vi "ArrayView.vi"(4 "Properties":T2={"Colormap"={"Map"=enum."Automatic", "Value Min"=nan, "Value Max"=nan, "Scaling"=enum."Default", "Reverse"=FALSE}, "Display"={"Alpha"=nan, "Z Order"=nan}}, 6 "Boundaries":T1={"X Min"=nan, "X Max"=nan, "Y Min"=nan, "Y Max"=nan}, 7 "Data":dbl[][](array[numeric]), 8 "error in (no error)":errorcluster, 11 "Plot ID":T7 format="%x") -> (0 "error out":errorcluster, 3 "Plot ID Out":T7 format="%x")   [LabVIEW 2013, in "Advanced Plotting Toolkit.lvlib"]
doc: "Display a 2D array as pseudocolor, using a colormap."
uses:
  Advanced Plotting Toolkit.lvlib
  typedefs/PlotID.ctl
  ArrayViewProperties.ctl
  properties/Colormap.ctl
  properties/Colormap_Map.ctl
  properties/Colormap_Scaling.ctl
  properties/Display.ctl
  ArrayViewBoundaries.ctl
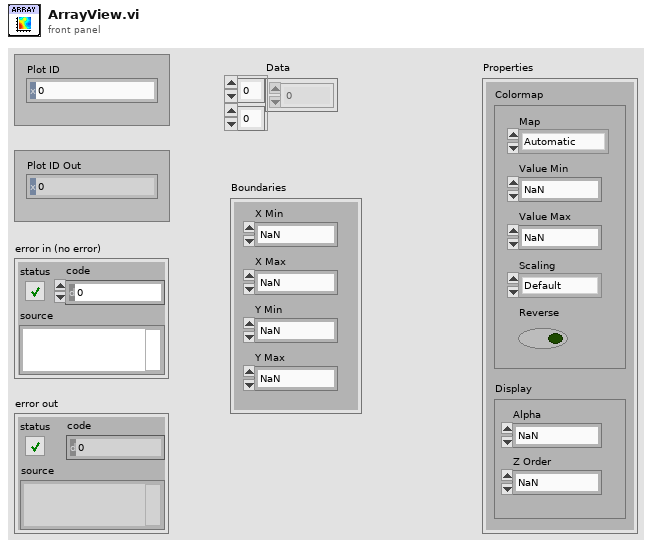
[diagram p1: front panel]
types:
  T1 = typedef "Advanced Plotting Toolkit.lvlib/ArrayViewBoundaries.ctl" = cluster{"X Min":dbl, "X Max":dbl, "Y Min":dbl, "Y Max":dbl}
  T2 = typedef "Advanced Plotting Toolkit.lvlib/ArrayViewProperties.ctl" = cluster{"Colormap":T3, "Display":T6}
  T3 = typedef "Advanced Plotting Toolkit.lvlib/Colormap.ctl" = cluster{"Map":T4, "Value Min":dbl, "Value Max":dbl, "Scaling":T5, "Reverse":bool}
  T4 = typedef "Advanced Plotting Toolkit.lvlib/Colormap_Map.ctl" = enum16{"Automatic", "Rainbow", "Hot and Cold", "White-Black", "White-Blue", "White-Green", "White-Red", "Fire", "Water", "Earth", "Air", "Pastel", "Banded", "Stepped"}
  T5 = typedef "Advanced Plotting Toolkit.lvlib/Colormap_Scaling.ctl" = enum16{"Default"}
  T6 = typedef "Advanced Plotting Toolkit.lvlib/Display.ctl" = cluster{"Alpha":dbl, "Z Order":dbl}
  T7 = typedef "Advanced Plotting Toolkit.lvlib/PlotID.ctl" = i32
  T8 = typedef "Advanced Plotting Toolkit.lvlib/KeyValue.ctl" = cluster{"Key":string, "Value":string}
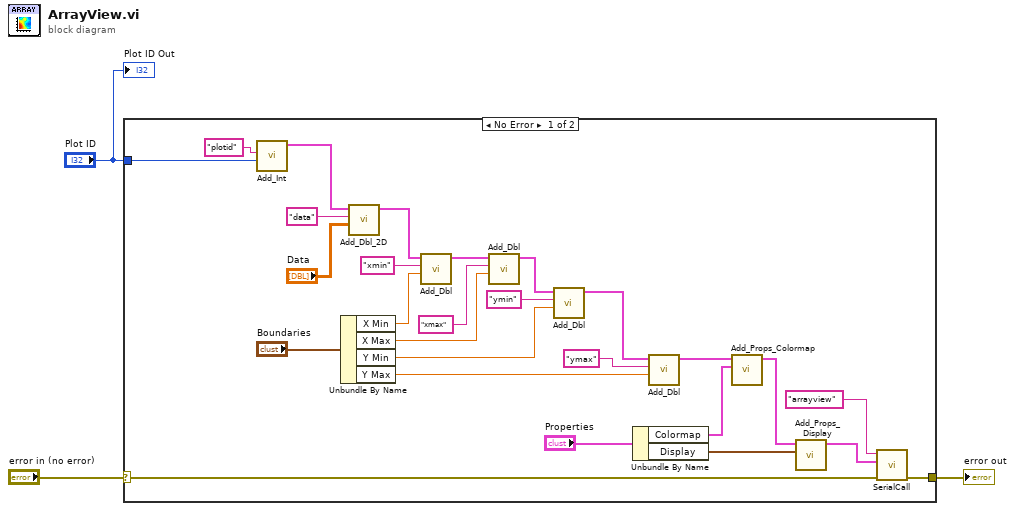
[diagram p0: block diagram]
diagram:
  n1 = case shown="No Error" "error in (no error)" {
    selector: "error in (no error)" -> [w28 w31]
    tunnel: "Plot ID" -> [w30 _]
    tunnel: [w27 w31] -> w1
    frame No Error {
      n2 = call "Add_Int.vi"("Value"=w30, "Key"="plotid") -> ("Keyword Array Out"=w26:T8[])  [unwired: 9 in]
      n3 = Unbundle By Name("Boundaries") -> ("X Min"=w7:dbl, "X Max"=w6:dbl, "Y Min"=w5:dbl, "Y Max"=w4:dbl)
      n4 = call "Add_Dbl_2D.vi"("Value"="Data", "Key"="data", "Keyword Array"=w26) -> ("Keyword Array Out"=w17:T8[])  [unwired: 8 in]
      n5 = call "Add_Dbl.vi"("Value"=w7, "Key"="xmin", "Keyword Array"=w17) -> ("Keyword Array Out"=w12:T8[])  [unwired: 8 in]
      n6 = call "Add_Dbl.vi"("Value"=w6, "Key"="xmax", "Keyword Array"=w12) -> ("Keyword Array Out"=w11:T8[])  [unwired: 8 in]
      n7 = call "Add_Dbl.vi"("Value"=w5, "Key"="ymin", "Keyword Array"=w11) -> ("Keyword Array Out"=w10:T8[])  [unwired: 8 in]
      n8 = Unbundle By Name("Properties") -> ("Colormap"=w22:T3, "Display"=w20:T6)
      n9 = call "Add_Dbl.vi"("Value"=w4, "Key"="ymax", "Keyword Array"=w10) -> ("Keyword Array Out"=w9:T8[])  [unwired: 8 in]
      n10 = call "Add_Props_Colormap.vi"("Colormap"=w22, "Keyword Array"=w9) -> ("Keyword Array Out"=w18:T8[])  [unwired: 9 in]
      n11 = call "Add_Props_Display.vi"("Display"=w20, "Keyword Array"=w18) -> ("Keyword Array Out"=w19:T8[])  [unwired: 9 in]
      n12 = call "SerialCall.vi"("error in (no error)"=w28, "data"=w19, "Resource"="arrayview") -> ("error out"=w27:errorcluster)  [unwired: 7 in, 1 out]
    }
    frame Error {
    }
  }
  "error out" <- w1
  "Plot ID Out" <- "Plot ID"
